vi "INIT.vi"(8 "error in (no error)":errorcluster, 11 "Soda Actor in":refnum<class "Soda Actor.lvclass">) -> (0 "error out":errorcluster, 3 "Soda Actor out":refnum<class "Soda Actor.lvclass">)   [LabVIEW 2020, in "Soda Actor.lvlib" / "Soda Actor.lvclass"]
uses:
  Soda Actor.lvclass
  Soda Actor.lvclass/Soda Actor.ctl
  <vilib>/Utility/config.llb/Read Key (Double).vi
  <vilib>/Utility/config.llb/Read Key (String).vi
  <vilib>/Utility/config.llb/NI_LVConfig.lvlib
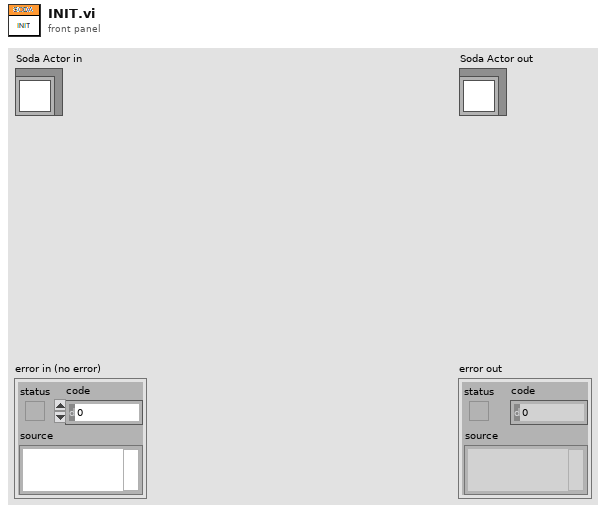
[diagram p1: front panel]
types:
  T1 = typedef "NI_LVConfig.lvlib/Config Data RefNum.ctl" = refnum<k1>
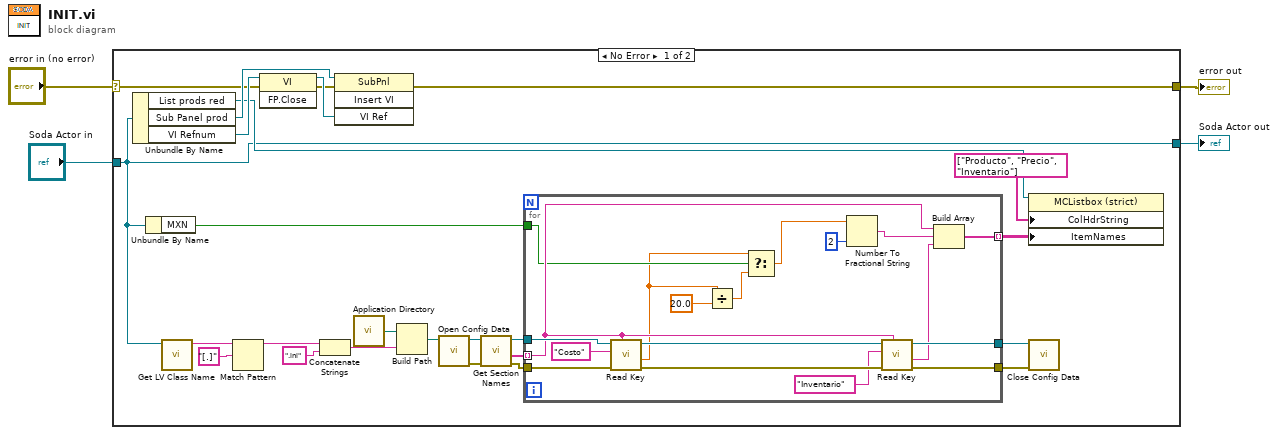
[diagram p0: block diagram]
diagram:
  n1 = case shown="No Error" "error in (no error)" {
    selector: "error in (no error)" -> [w24 w48]
    tunnel: [w12 w49] -> w2
    tunnel: "Soda Actor in" -> [w12 w49]
    tunnel: [w25 w48] -> w1
    frame No Error {
      n2 = Unbundle By Name(w12) -> ("List prods red"=w23:refnum<vi>, "Sub Panel prod"=w29:refnum<vi>, "VI Refnum"=w28:refnum<vi>)
      n3 = Unbundle By Name(w12) -> ("MXN"=w11:bool)
      n4 = call <vilib>:"Get LV Class Name.vi"("object"=w12) -> ("class name"=w14:string)  [unwired: 9 in, 1 out]
      n5 = Match Pattern(string=w14, regular expression="[.]") -> (before substring=w5:string)  [unwired: 1 in, 3 out]
      n6 = invoke class="VI" method="FP.Close"(reference=w28, error in=w24) -> (reference out=w27:refnum<vi>, error out=w26:errorcluster)  [unwired: 1 in, 1 out]
      n7 = Concatenate Strings(w5, ".ini" ("string")) -> (w20:string)
      n8 = invoke class="SubPnl" method="Insert VI"(reference=w29, error in=w26, "VI Ref"=w27) -> (error out=w25:errorcluster)  [unwired: 1 in, 3 out]
      n9 = call <vilib>:"Application Directory.vi"() -> ("Application Directory"=w19:path)
      n10 = Build Path(base path=w19, name or relative path=w20) -> (appended path=w18:path)
      n11 = call <vilib>:"Open Config Data.vi"("configuration file path"=w18) -> ("error out"=w17:errorcluster, "refnum"=w9:T1)  [unwired: 8 in, 1 out]
      n12 = call <vilib>:"Get Section Names.vi"("error in (no error)"=w17, "refnum"=w9) -> ("error out"=w10:errorcluster, "section names"=w7:string[], "refnum out"=w8:T1)  [unwired: 7 in]
      n13 = for {
        tunnel: w8 -> [w47]
        tunnel: w10 -> [w46]
        tunnel: [w43] -> w16
        tunnel: [w42] -> w15
        tunnel: w11 -> [w34]
        tunnel: w7 -> [w39] mode=indexing
        tunnel: [w37] -> w6 mode=indexing
        n14 = call-poly <vilib>:"Read Key.vi"("section"=w39, "error in (no error)"=w46, "key"="Costo", "refnum"=w47) -> ("error out"=w45:errorcluster, "value"=w32:dbl, "refnum out"=w44:T1)  [unwired: 4 in, 1 out]
        n15 = Divide(x=w32, y=20.0) -> (x/y=w30:dbl)
        n16 = Select(t=w32, s=w34, f=w30) -> (s? t:f=w33:dbl)
        n17 = Number To Fractional String(number=w33, precision (6)=i16 2) -> (F-format string=w36:string)  [unwired: 2 in]
        n18 = call-poly <vilib>:"Read Key.vi"("section"=w39, "error in (no error)"=w45, "key"="Inventario", "refnum"=w44) -> ("error out"=w43:errorcluster, "value"=w38:string, "refnum out"=w42:T1)  [unwired: 4 in, 1 out]
        n19 = Build Array(w39, w36, w38) -> (w37:string[])
      }
      n20 = property class="MCListbox (strict)"(reference=w23, "ColHdrString"=string[] ["Producto", "Precio", "Inventario"] ("Column Header Strings[]"), "ItemNames"=w6) -> ()  [unwired: 1 in, 2 out]
      n21 = call <vilib>:"Close Config Data.vi"("error in (no error)"=w16, "refnum"=w15) -> ()  [unwired: 8 in, 2 out]
    }
    frame Error {
    }
  }
  "error out" <- w1
  "Soda Actor out" <- w2
